vi "PowerSetup.vi"(8 "Current limit heater":dbl=1.0, 9 "bias Pt100":dbl=5.0 caption="Voltage (0.0)" format="%^.3e", 10 "Current limit Pt100":dbl=0.1 caption="Current (0.0)" format="%.3p", 11 "VISA resource name":refnum<visa-resource-name>="USB0::0x0AAD::0x0135::034083383::INSTR") -> (0 "error out":errorcluster, 3 "VISA resource name out":refnum<visa-resource-name>)   [LabVIEW 2014]
uses:
  <instrlib>/Rohde&Schwarz HMC 804x Power Supplies/Rohde&Schwarz HMC 804x Power Supplies.lvlib
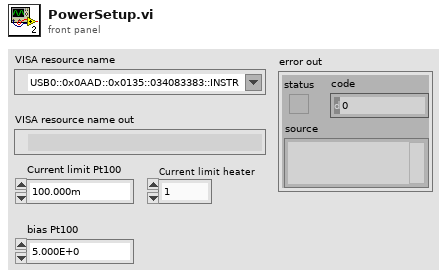
[diagram p1: front panel]
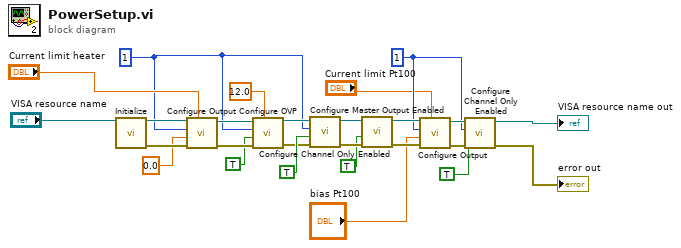
[diagram p0: block diagram]
diagram:
  w14 = 1 ("Channel (1)")
  w3 = 1 ("Channel (1)")
  n1 = call <instrlib>:"Initialize.vi"("VISA resource name"="VISA resource name") -> ("VISA resource name out"=w23:refnum<visa-resource-name>, "error out"=w24:errorcluster)  [unwired: 13 in]
  n2 = call <instrlib>:"Configure Output.vi"("Current (0.0)"="Current limit heater", "error in (no error)"=w24, "Voltage (0.0)"=0.0, "Channel (1)"=w3, "VISA resource name"=w23) -> ("error out"=w6:errorcluster, "VISA resource name out"=w7:refnum<visa-resource-name>)  [unwired: 5 in]
  n3 = call <instrlib>:"Configure OVP.vi"("Limit (0.0)"=12.0, "error in (no error)"=w6, "Enabled (Off)"=TRUE, "Channel (1)"=w3, "VISA resource name"=w7) -> ("error out"=w5:errorcluster, "VISA resource name out"=w4:refnum<visa-resource-name>)  [unwired: 5 in]
  n4 = call <instrlib>:"Configure Channel Only Enabled.vi"("error in (no error)"=w5, "Enabled (Off)"=TRUE, "Channel (1)"=w3, "VISA resource name"=w4) -> ("error out"=w26:errorcluster, "VISA resource name out"=w25:refnum<visa-resource-name>)  [unwired: 6 in]
  n5 = call <instrlib>:"Configure Master Output Enabled.vi"("error in (no error)"=w26, "Enabled (Off)"=TRUE, "VISA resource name"=w25) -> ("error out"=w18:errorcluster, "VISA resource name out"=w19:refnum<visa-resource-name>)  [unwired: 7 in]
  n6 = call <instrlib>:"Configure Output.vi"("Current (0.0)"="Current limit Pt100", "error in (no error)"=w18, "Voltage (0.0)"="bias Pt100", "Channel (1)"=w14, "VISA resource name"=w19) -> ("error out"=w21:errorcluster, "VISA resource name out"=w20:refnum<visa-resource-name>)  [unwired: 5 in]
  n7 = call <instrlib>:"Configure Channel Only Enabled.vi"("error in (no error)"=w21, "Enabled (Off)"=TRUE, "Channel (1)"=w14, "VISA resource name"=w20) -> ("error out"=→"error out":errorcluster, "VISA resource name out"=→"VISA resource name out":refnum<visa-resource-name>)  [unwired: 6 in]
